vi "Stop Devices.vi"(8 "error in (no error)":errorcluster, 11 "Device Manager in":refnum<class "Device Manager.lvclass">) -> (0 "error out":errorcluster, 3 "Device Manager out":refnum<class "Device Manager.lvclass">)   [LabVIEW 2023, in "Device Manager.lvclass"]
uses:
  Device Manager.lvclass
  Device Manager.lvclass/Device Manager.ctl
  Device/Device Messages/Stop Action Msg/Stop Action Msg.lvclass
  Device/Device Messages/Clear Action Msg/Clear Action Msg.lvclass
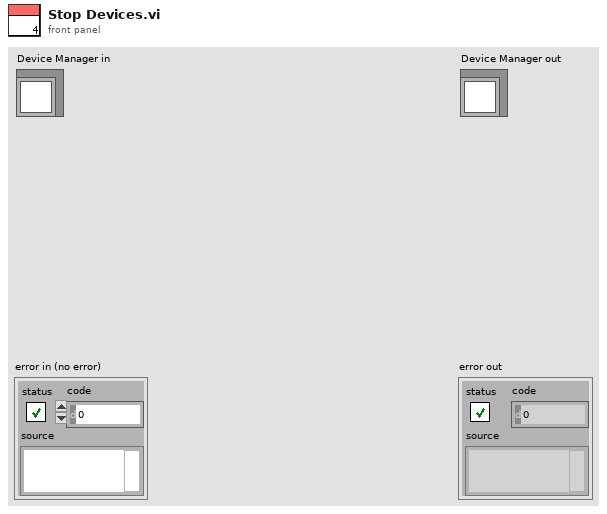
[diagram p1: front panel]
types:
  T1 = map{string, refnum<class "Message Enqueuer.lvclass">}
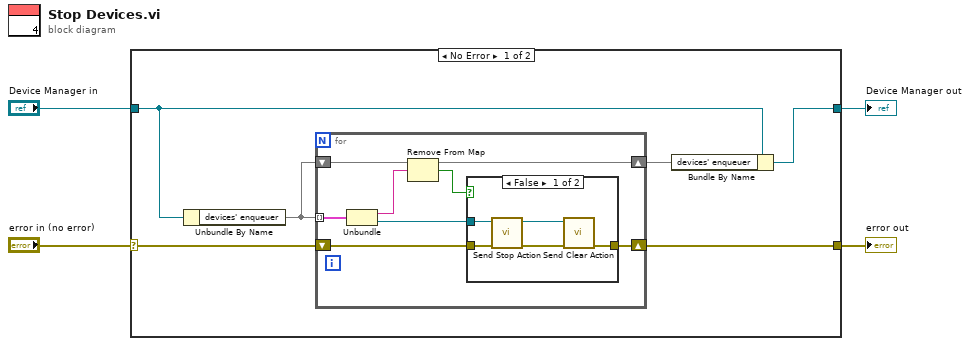
[diagram p0: block diagram]
diagram:
  n1 = case shown="No Error" "error in (no error)" {
    selector: "error in (no error)" -> [w10 w26]
    tunnel: [w9 w26] -> w3
    tunnel: [w5 w25] -> w1
    tunnel: "Device Manager in" -> [w7 w25]
    frame No Error {
      n2 = Unbundle By Name(w7) -> ("devices' enqueuer"=w8:T1)
      n3 = for {
        tunnel: w8 -> [w15] mode=indexing
        shift-right: [w17] -> w9
        shift-left: w10 -> [w18]
        shift-right: [w12] -> w6
        shift-left: w8 -> [w16]
        n4 = Unbundle(w15) -> ("device"=w13:string, "enqueuer"=w14:refnum<class "Message Enqueuer.lvclass">)
        n5 = Remove From Map(10:w13, 11:w16) -> (2:w11:bool, 3:w12:T1)  [unwired: 1 out]
        n6 = case shown="False" w11 {
          tunnel: w18 -> [w21 w24]
          tunnel: [w20 w24] -> w17
          tunnel: w14 -> [w19 _]
          frame False {
            n7 = call "Send Stop Action.vi"("error in (no error)"=w21, "Message Enqueuer"=w19) -> ("error out"=w23:errorcluster, "Message Enqueuer out"=w22:refnum<class "Message Enqueuer.lvclass">)  [unwired: 8 in]
            n8 = call "Send Clear Action.vi"("error in (no error)"=w23, "Message Enqueuer"=w22) -> ("error out"=w20:errorcluster)  [unwired: 8 in, 1 out]
          }
          frame True {
          }
        }
      }
      n9 = Bundle By Name(cluster=w7, "devices' enqueuer"=w6) -> (w5:refnum<class "Device Manager.lvclass">)
    }
    frame Error {
    }
  }
  "error out" <- w3
  "Device Manager out" <- w1
